vi "Single Acquisition (Amplitude Reg) UI.vi"() -> ()   [LabVIEW 2014]
uses:
  <vilib>/FPGAPlugInAG/sbRIO-9636/niLvFpga_Open_sbRIO-9636.vi
  <vilib>/rvi/interface/common/dynamic/niFpgaDynamicAddResources.vi
  <vilib>/Utility/error.llb/Error Cluster From Error Code.vi
  <vilib>/rvi/errors/niLvFpgaAdjustHostInterfaceError.vi
  <vilib>/rvi/interface/common/niFpgaWaitOnOcc.vi
  <vilib>/FPGAPlugInAG/Dynamic/niLvFpga_Run_Dynamic.vi
  <vilib>/FPGAPlugInAG/Dynamic/niLvFpga_Close_Dynamic.vi
  <vilib>/rvi/interface/nirviOpenFPGA/nirviOpenFPGA.xnode
  FPGA Bitfiles/LaserDistanceSen_FPGATarget_Acquisition&Gene_n7KIVm0uJjs.lvbitx
  <vilib>/rvi/interface/nirviReadWriteControl/nirviReadWriteControl.xnode
  <vilib>/rvi/interface/nirviMethod/nirviMethod.xnode
  <vilib>/rvi/interface/nirviCloseFPGA/nirviCloseFPGA.xnode
  <vilib>/rvi/errors/niLvFpgaMergeErrorWithErrorCode.vi
  <vilib>/FPGAPlugInAG/Dynamic/niLvFpga_ConfigureFifo_Dynamic.vi
  <vilib>/FPGAPlugInAG/Dynamic/niLvFpga_StartFifo_Dynamic.vi
  <vilib>/FPGAPlugInAG/Dynamic/niLvFpga_ReadFifo_Dynamic.vi
  NiFpgaLv.dll
  <vilib>/rvi/interface/Simulation/niFpgaSimulationCallBeginRW.vi
panel:
  in  "Amplitude (0:1)":fxp<+,4,1>
  in  "Number of Elements to read":u32=512
  out "Waveform Graph (input data)":dbl[](graph)
  out "Elements Remaining":u32
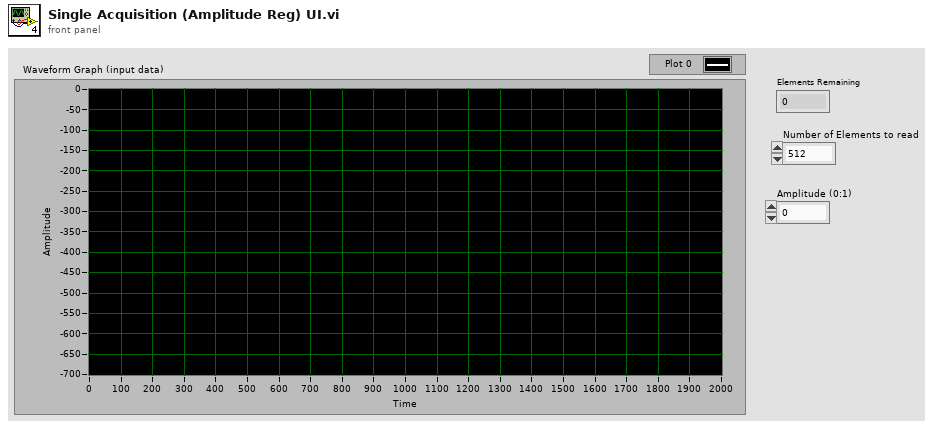
[diagram p1: front panel]
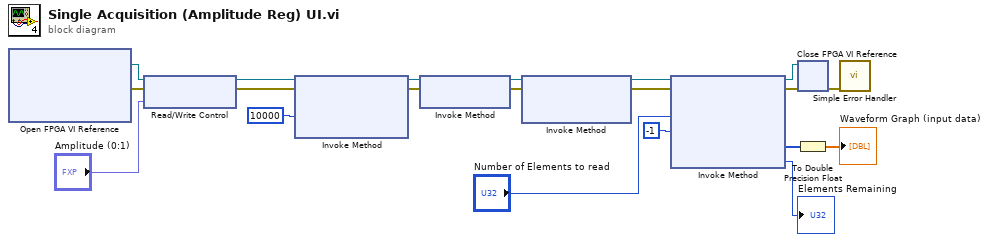
[diagram p0: block diagram]
diagram:
  n1 = xnode "Open FPGA VI Reference"() -> ("FPGA VI Reference Out"=w7:refnum<k20>, "error out"=w6:errorcluster)  [unwired: 2 in]
  n2 = xnode "Read/Write Control"("FPGA VI Reference In"=w7, "error in"=w6, "Amplitude (0:1)"="Amplitude (0:1)") -> ("FPGA VI Reference Out"=w5:refnum<k20>, "error out"=w4:errorcluster)
  n3 = xnode "Invoke Method"("FPGA VI Reference In"=w5, "error in"=w4, "Requested Depth"=u32 10000) -> ("FPGA VI Reference Out"=w18:refnum<k20>, "error out"=w19:errorcluster)  [unwired: 1 out]
  n4 = xnode "Invoke Method"("FPGA VI Reference In"=w18, "error in"=w19) -> ("FPGA VI Reference Out"=w16:refnum<k20>, "error out"=w17:errorcluster)
  n5 = xnode "Invoke Method"("FPGA VI Reference In"=w16, "error in"=w17) -> ("FPGA VI Reference Out"=w2:refnum<k20>, "error out"=w3:errorcluster)  [unwired: 1 in]
  n6 = xnode "Invoke Method"("FPGA VI Reference In"=w2, "error in"=w3, "Number of Elements"="Number of Elements to read", "Timeout (ms)"=-1) -> ("FPGA VI Reference Out"=w14:refnum<k20>, "error out"=w13:errorcluster, "Data"=w9:i16[], "Elements Remaining"=→"Elements Remaining":u32)
  n7 = xnode "Close FPGA VI Reference"("FPGA VI Reference In"=w14, "error in"=w13) -> ("error out"=w15:errorcluster)
  n8 = To Double Precision Float(number=w9) -> (double precision float=→"Waveform Graph (input data)":dbl[])
  n9 = call <vilib>:"Simple Error Handler.vi"("error in (no error)"=w15) -> ()  [unwired: 4 in, 5 out]
